vi "Rogowski_Coil_Correction_FreqDomain.vi"(4 "Phase change(Deg)":dbl=90.0, 6 "HighPass\nFreq":dbl=500.0, 7 "Freq array":dbl[](array[numeric])=array[31500 elements], 11 "Raw IMon FFT":T1={"f0"=0.0, "df"=15.873015873016348, "magnitude"=array[31500 elements], "phase"=array[31500 elements], "PSD"=array[31500 elements]}) -> (2 "Corrected Amplitude":dbl[](array[numeric]), 3 "TF Corr IMon FFT":T1={"f0"=0.0, "df"=15.873015873016348, "magnitude"=array[31500 elements], "phase"=array[31500 elements], "PSD"=array[31500 elements]})   [LabVIEW 2021]
uses:
  MPS_Labview/MPS_global_variables.vi
panel:
  out "Waveform Graph":cluster{"f0":dbl, "df":dbl, "magnitude":dbl[]}(graph)
  out "Corrected FFT":cluster{"f0":dbl, "df":dbl, "magnitude":dbl[]}(graph)={"f0"=0.0, "df"=17.006802721088945, "magnitude"=array[29400 elements]}
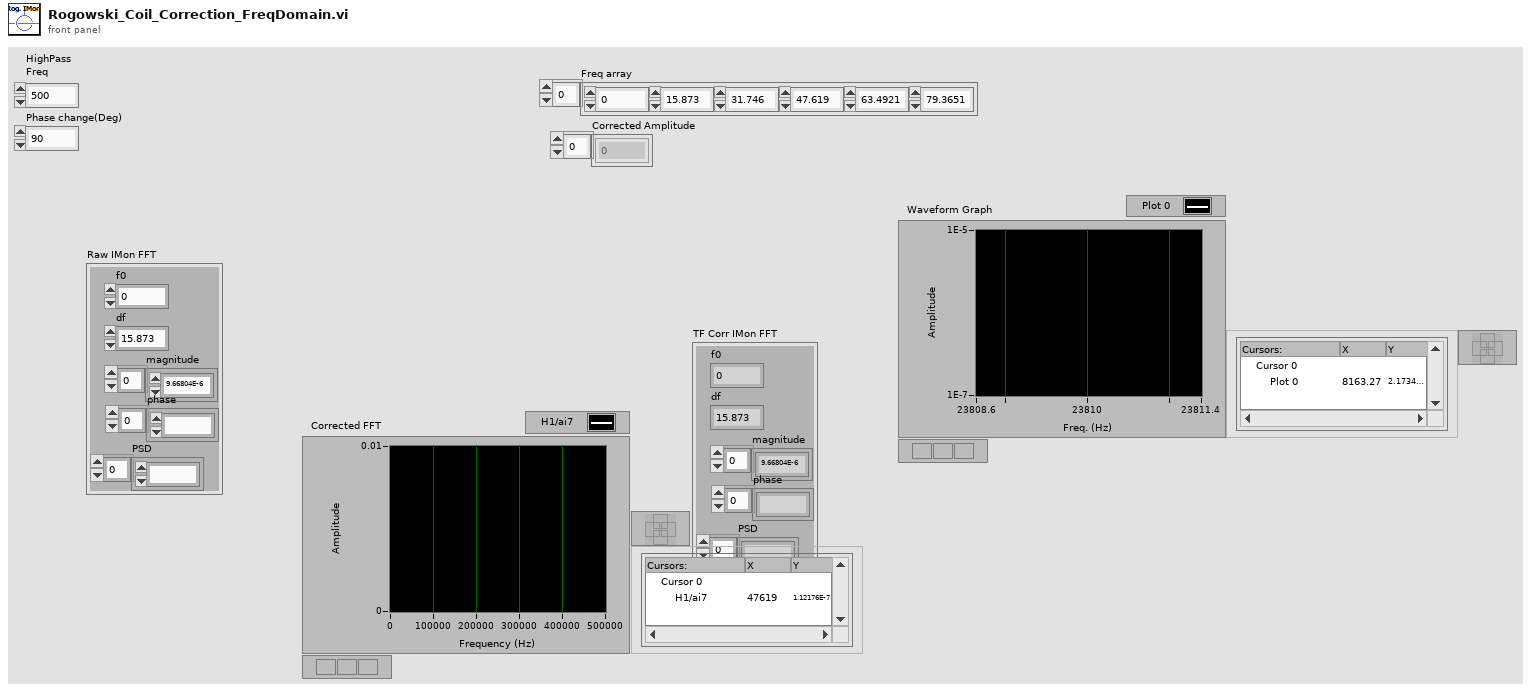
[diagram p1: front panel]
types:
  T1 = cluster{"f0":dbl, "df":dbl, "magnitude":dbl[], "phase":dbl[], "PSD":dbl[]}
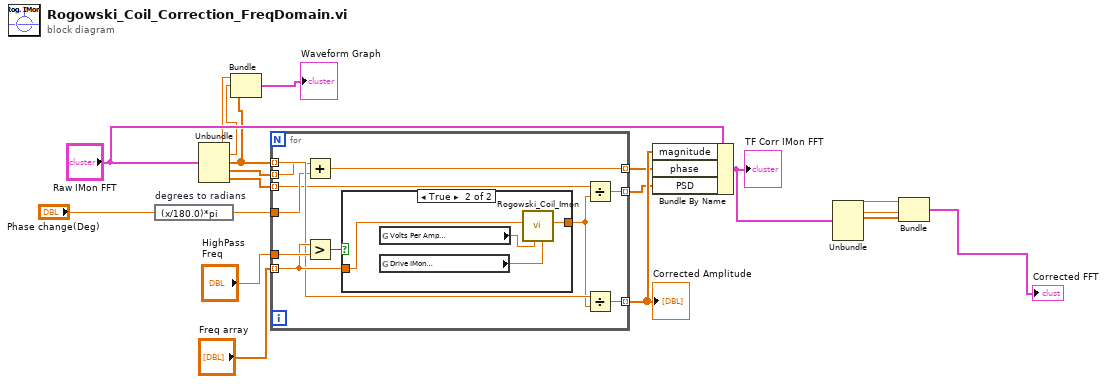
[diagram p0: block diagram]
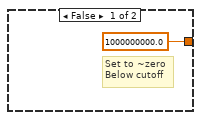
[diagram p2: hidden frame]
diagram:
  n1 = expression code="(x/180.0)*pi" "degrees to radians"("Phase change(Deg)") -> (w14:dbl)
  n2 = Unbundle("Raw IMon FFT") -> ("f0"=w4:dbl, "df"=w3:dbl, "magnitude"=w2:dbl[], "phase"=w19:dbl[], "PSD"=w18:dbl[])
  n3 = Bundle("f0"=w4, "df"=w3, "magnitude"=w2) -> (→"Waveform Graph":cluster{"f0":dbl, "df":dbl, "magnitude":dbl[]})  [unwired: 1 in]
  n4 = for {
    tunnel: w2 -> [w27] mode=indexing
    tunnel: w19 -> [w26] mode=indexing
    tunnel: w18 -> [w24] mode=indexing
    tunnel: "HighPass\nFreq" -> [w30]
    tunnel: "Freq array" -> [w28] mode=indexing
    tunnel: w14 -> [w25]
    tunnel: [w22] -> w12 mode=indexing
    tunnel: [w21] -> w11 mode=indexing
    tunnel: [w20] -> w10 mode=indexing
    n5 = Add(x=w26, y=w25) -> (x+y=w21:dbl)
    n6 = Greater?(x=w28, y=w30) -> (0:w29:bool)
    n7 = case shown="True" w29 {
      tunnel: w28 -> [_ w35]
      tunnel: [1000000000.0 ("x*y") w32] -> w23
      frame False {
        # "Set to ~zero\nBelow cutoff"
      }
      frame True {
        n8 = global read "MPS_global_variables.vi" "Volts Per Amp\nDrive"() -> (w33:dbl)
        n9 = global read "MPS_global_variables.vi" "Drive IMon\nRef Freq"() -> (w34:dbl)
        n10 = call "Rogowski_Coil_Imon.vi"("Ref_Freq"=w34, "RefGain"=w33, "CurrentFreq"=w35) -> ("x*y"=w32:dbl)  [unwired: 8 in]
      }
    }
    n11 = Divide(x=w24, y=w23) -> (x/y=w20:dbl)
    n12 = Divide(x=w27, y=w23) -> (x/y=w22:dbl)
  }
  "Corrected Amplitude" <- w12
  n13 = Bundle By Name(cluster="Raw IMon FFT", "magnitude"=w12, "phase"=w11, "PSD"=w10) -> (w9:T1)
  "TF Corr IMon FFT" <- w9
  n14 = Unbundle(w9) -> ("f0"=w8:dbl, "df"=w7:dbl, "magnitude"=w6:dbl[])  [unwired: 2 out]
  n15 = Bundle("f0"=w8, "df"=w7, "magnitude"=w6) -> (→"Corrected FFT":cluster{"f0":dbl, "df":dbl, "magnitude":dbl[]})  [unwired: 1 in]
